vi "1553 Channels to Channel Handles.vi"(8 "error in":errorcluster, 10 "1553 channels":T5[](array[typedef]), 11 "Ballard MIL-STD 1553 custom device in":T4 format="%.0x") -> (0 "error out":errorcluster, 1 "Tx Channels":T4[](array[typedef]) format="%.0x", 2 "Rx Channels":T4[](array[typedef]) format="%.0x", 3 "Ballard MIL-STD 1553 custom device out":T4 format="%.0x", 4 "1553 channel handles":T1[](array[typedef]) {"messages"."timestamps" format="%.0x"; "messages"."parameters"."RxBC channel handle" format="%.0x"; "messages"."parameters"."RxRT channel handle" format="%.0x"; "messages"."parameters"."Tx channel handle" format="%.0x"})   [LabVIEW 2020, in "Ballard MIL-STD-1553 Engine.lvlib" / "Implementation.lvlib" / "Execution Unit.lvclass"]
uses:
  Execution Unit.lvclass
  <vilib>/NI VeriStand/Custom Device API/Custom Device Item Ref.ctl
  <vilib>/NI VeriStand/Custom Device API/Custom Device API.lvlib
  1553 Channel Handles.ctl
  Scripting/Ballard MIL-STD-1553 Scripting.lvlib
  Parameter Handles.ctl
  Message Handles.ctl
  Shared/Address.ctl
  Shared/Terminal Endpoint.ctl
  Shared/Parameter Definition.ctl
  Shared/Message Type.ctl
  Shared/Message Definition.ctl
  Shared/Terminal Name and Address.ctl
  Shared/1553 Channel.ctl
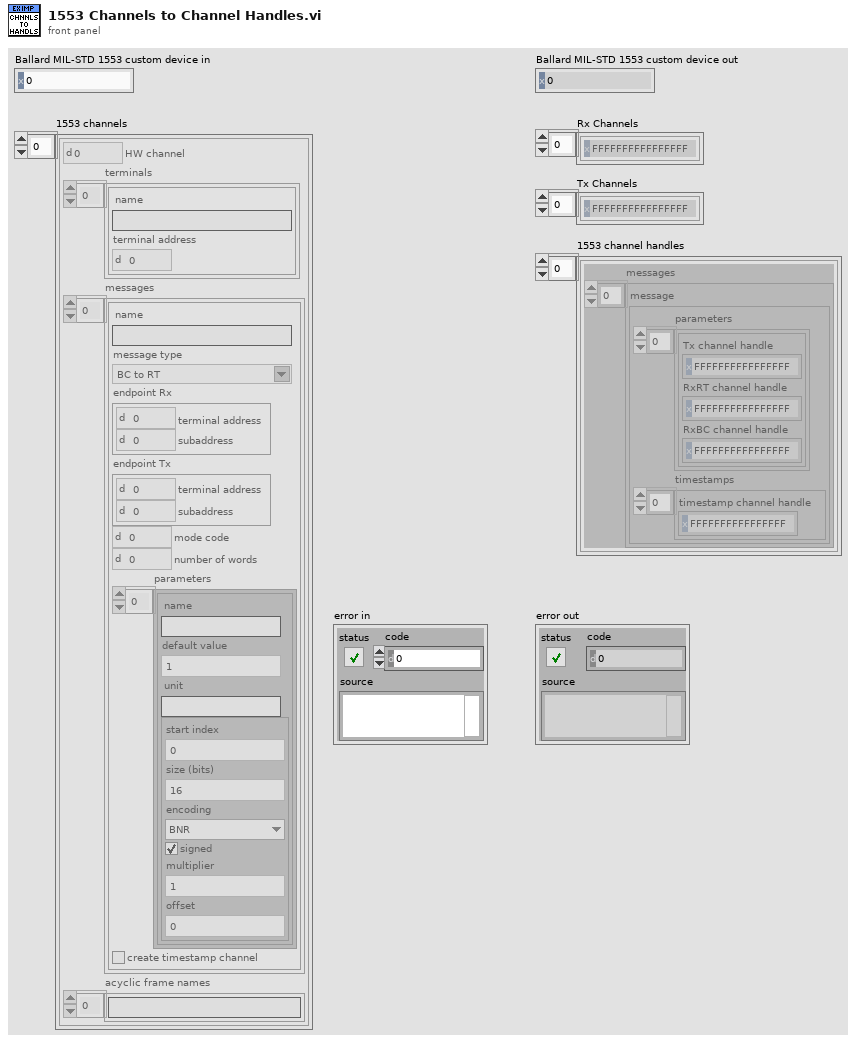
[diagram p1: front panel]
types:
  T1 = typedef "Ballard MIL-STD-1553 Engine.lvlib/Implementation.lvlib/Execution Unit.lvclass/1553 Channel Handles.ctl" = cluster{"messages":T2[]}
  T2 = typedef "Ballard MIL-STD-1553 Engine.lvlib/Implementation.lvlib/Execution Unit.lvclass/Message Handles.ctl" = cluster{"parameters":T3[], "timestamps":T4[]}
  T3 = typedef "Ballard MIL-STD-1553 Engine.lvlib/Implementation.lvlib/Execution Unit.lvclass/Parameter Handles.ctl" = cluster{"Tx channel handle":T4, "RxRT channel handle":T4, "RxBC channel handle":T4}
  T4 = typedef "Custom Device API.lvlib/Custom Device Item Ref.ctl" = u64
  T5 = typedef "1553 Channel.ctl" = cluster{"HW channel":u16, "terminals":T6[], "messages":T8[], "acyclic frame names":string[]}
  T6 = typedef "Terminal Name and Address.ctl" = cluster{"name":string, "terminal address":T7}
  T7 = typedef "Address.ctl" = u16
  T8 = typedef "Message Definition.ctl" = cluster{"name":string, "message type":T9, "endpoint Rx":T10, "endpoint Tx":T10, "mode code":u16, "number of words":u16, "parameters":cluster{"name":string, "default value":dbl, "unit":string, "parameter definition":T11}[], "create timestamp channel":bool}
  T9 = typedef "Message Type.ctl" = string
  T10 = typedef "Terminal Endpoint.ctl" = cluster{"terminal address":T7, "subaddress":T7}
  T11 = typedef "Parameter Definition.ctl" = cluster{"start index":i32, "size (bits)":i32, "encoding":enum16{"BNR", "BCD", "Discrete"}, "signed":bool, "multiplier":dbl, "offset":dbl}
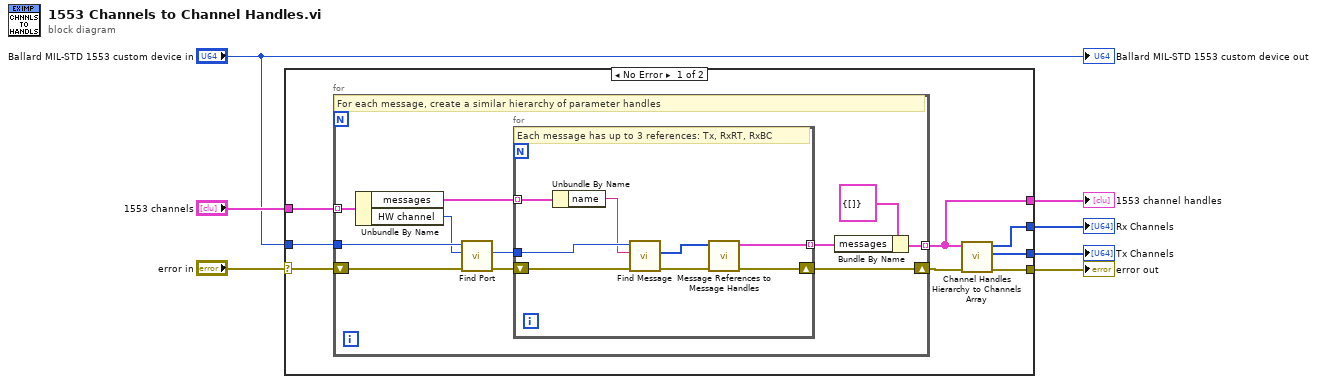
[diagram p0: block diagram]
diagram:
  n1 = case shown="No Error" "error in" {
    selector: "error in" -> [w14 w35]
    tunnel: "1553 channels" -> [w15 _]
    tunnel: "Ballard MIL-STD 1553 custom device in" -> [w13 _]
    tunnel: [w11 w35] -> w5
    tunnel: [w10 _] -> w4
    tunnel: [w9 _] -> w3
    tunnel: [w8 _] -> w1
    frame No Error {
      n2 = for {
        tunnel: w15 -> [w26] mode=indexing
        shift-right: [w16] -> w12
        shift-left: w14 -> [w25]
        tunnel: w13 -> [w24]
        tunnel: [w17] -> w8 mode=indexing
        # "For each message, create a similar hierarchy of parameter handles"
        n3 = Unbundle By Name(w26) -> ("messages"=w21:T8[], "HW channel"=w23:u16)
        n4 = call "Find Port.vi"("error in"=w25, "port number"=w23, "Ballard MIL-STD 1553 custom device in"=w24) -> ("error out"=w22:errorcluster, "port"=w20:T4)  [unwired: 5 in, 2 out]
        n5 = for {
          tunnel: w21 -> [w33] mode=indexing
          shift-right: [w28] -> w16
          shift-left: w22 -> [w34]
          tunnel: w20 -> [w32]
          tunnel: [w27] -> w18 mode=indexing
          # "Each message has up to 3 references: Tx, RxRT, RxBC"
          n6 = Unbundle By Name(w33) -> ("name"=w31:string)
          n7 = call "Find Message.vi"("error in"=w34, "message name"=w31, "port in"=w32) -> ("error out"=w30:errorcluster, "message refs"=w29:T4[])  [unwired: 5 in, 2 out]
          n8 = call "Message References to Message Handles.vi"("error in"=w30, "message refs"=w29) -> ("error out"=w28:errorcluster, "message handles"=w27:T2)  [unwired: 8 in]
        }
        n9 = Bundle By Name(cluster=T1 {"messages"=[]} ("1553 channel handles"), "messages"=w18) -> (w17:T1)
      }
      n10 = call "Channel Handles Hierarchy to Channels Array.vi"("error in"=w12, "1553 channel handles"=w8) -> ("error out"=w11:errorcluster, "Tx Channels"=w10:T4[], "Rx Channels"=w9:T4[])  [unwired: 7 in]
    }
    frame Error {
    }
  }
  "Rx Channels" <- w3
  "error out" <- w5
  "Tx Channels" <- w4
  "1553 channel handles" <- w1
  "Ballard MIL-STD 1553 custom device out" <- "Ballard MIL-STD 1553 custom device in"
